vi "libssh2_agent_publickey_refnum_delete.vi"(8 "error in (no error)":errorcluster, 11 "public key":T1) -> (0 "error out":errorcluster, 3 "libssh2_agent_publickey*":u64)   [LabVIEW 2013, in "libssh2.lvlib"]
doc: "Deletes <B>public key</B> and returns the associated pointer to libssh2_agent_publickey."
uses:
  libssh2.lvlib
  libssh2_agent_publickey_refnum.ctl
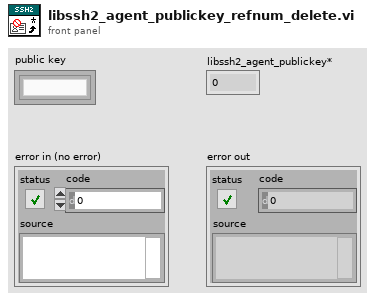
[diagram p1: front panel]
types:
  T1 = typedef "libssh2.lvlib/libssh2_agent_publickey_refnum.ctl" = refnum<k1>
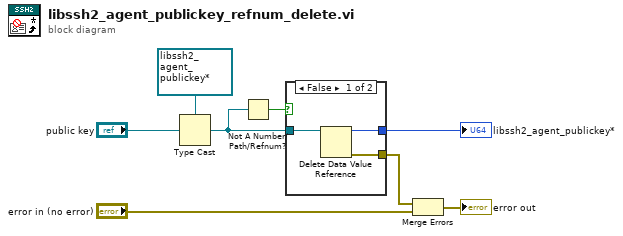
[diagram p0: block diagram]
diagram:
  n1 = Type Cast(type=refnum<data-value> refnum ("data value reference"), x="public key") -> (*(type *) &x=w5:refnum<data-value>)
  n2 = Not A Number/Path/Refnum?(number/path/refnum=w5) -> (NaN/Path/Refnum?=w4:bool)
  n3 = case shown="False" w4 {
    tunnel: [w11 _] -> w7
    tunnel: [w10 _] -> w6
    tunnel: w5 -> [w9 _]
    frame False {
      n4 = Delete Data Value Reference(data value reference=w9) -> (data value=w11:u64, error out=w10:errorcluster)  [unwired: 1 in]
    }
    frame True {
    }
  }
  "libssh2_agent_publickey*" <- w7
  n5 = Merge Errors(w6, "error in (no error)") -> (→"error out":errorcluster)
